vi "LJM_eReadNameByteArray.vi"(0 "Handle In":i32, 5 "Name":string, 11 "error in":errorcluster, 13 "NumBytes":i32) -> (4 "Handle Out":i32, 8 "aBytes":string, 14 "ErrorAddress":i32, 15 "error out":errorcluster)   [LabVIEW 2020]
uses:
  Library/Frameworks/LabJackM.framework
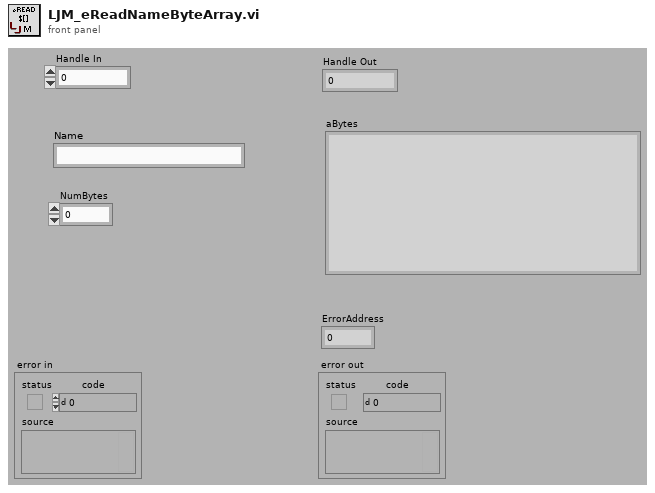
[diagram p1: front panel]
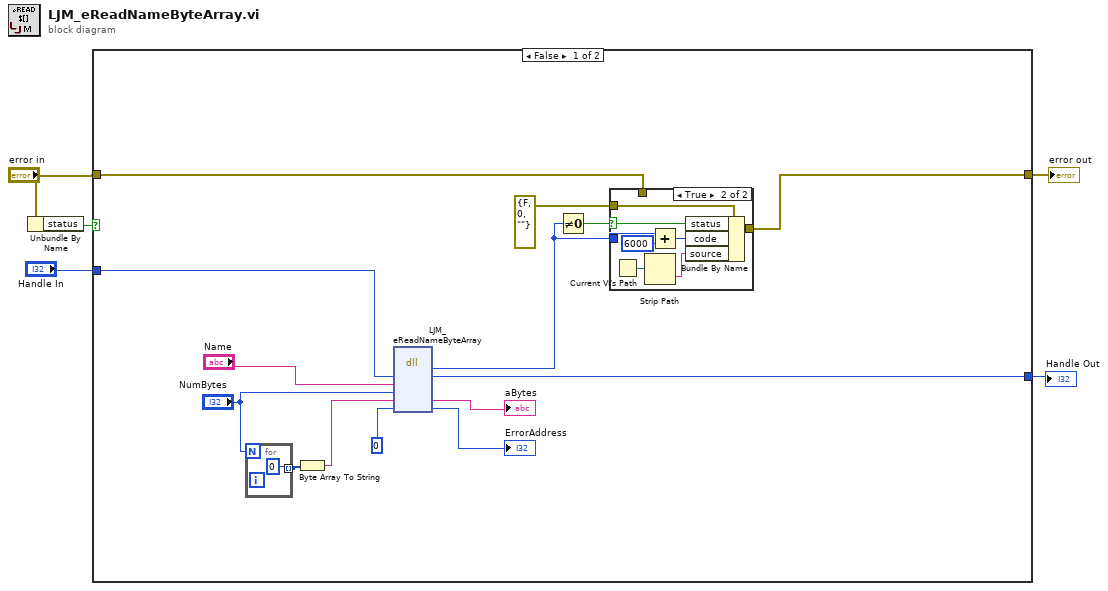
[diagram p0: block diagram]
diagram:
  n1 = Unbundle By Name("error in") -> ("status"=w5:bool)
  n2 = case shown="False" w5 {
    tunnel: "error in" -> [w16 w31]
    tunnel: [w15 w31] -> w2
    tunnel: [w14 w30] -> w1
    tunnel: "Handle In" -> [w13 w30]
    frame False {
      n3 = for {
        N: "NumBytes" -> [_]
        tunnel: [u8 0] -> w8 mode=indexing
      }
      n4 = Byte Array To String(unsigned byte array=w8) -> (string=w7:string)
      n5 = dll-call lib="Library/Frameworks/LabJackM.framework" fn="LJM_eReadNameByteArray"("Handle"=w13, "Name"="Name", "NumBytes"="NumBytes", "aBytes"=w7, "ErrorAddress"=u32 0 ("ErrorFrame")) -> ("return type"=w19:i32, "Handle"=w14:i32, "aBytes"=→"aBytes":string, "ErrorAddress"=→"ErrorAddress":i32)  [unwired: 5 in, 2 out]
      n6 = Not Equal To 0?(x=w19) -> (x != 0?=w18:bool)
      n7 = case shown="True" w18 {
        selector: w18 -> [_ w28]
        tunnel: [w21 w29] -> w15
        tunnel: errorcluster {"status"=FALSE, "code"=0, "source"=""} ("error IO") -> [_ w27]
        tunnel: w19 -> [_ w23]
        tunnel: w16 -> [w21 _]
        frame False {
        }
        frame True {
          n8 = Current VI's Path() -> (path=w25:path)
          n9 = Strip Path(path=w25) -> (name=w26:string)  [unwired: 1 out]
          n10 = Add(x=w23, y=6000) -> (x+y=w24:i32)
          n11 = Bundle By Name(cluster=w27, "status"=w28, "code"=w24, "source"=w26) -> (w29:errorcluster)
        }
      }
    }
    frame True {
    }
  }
  "error out" <- w2
  "Handle Out" <- w1
